vi "FileConfigDTOFromNative.vi"(8 "error in (no error)":errorcluster, 11 "FileConfig":T1={"rootFolder"=path "", "maxFileSize"=-1, "maxFileCount"=-1, "baseName"="", "extension"="", "delimiter"="", "calendarFolderTree"=FALSE}) -> (0 "error out":errorcluster, 3 "FileConfigDTO":T2={"rootFolder"="", "maxFileSize"=-1, "maxFileCount"=-1, "baseName"="", "extension"="", "delimiter"="", "calendarFolderTree"=FALSE})   [LabVIEW 2026, in "Lumberjack.lvlib"]
uses:
  Lumberjack.lvlib
  TypeDefs/ConfigDTO/FileConfigDTO.ctl
  TypeDefs/FileConfig.ctl
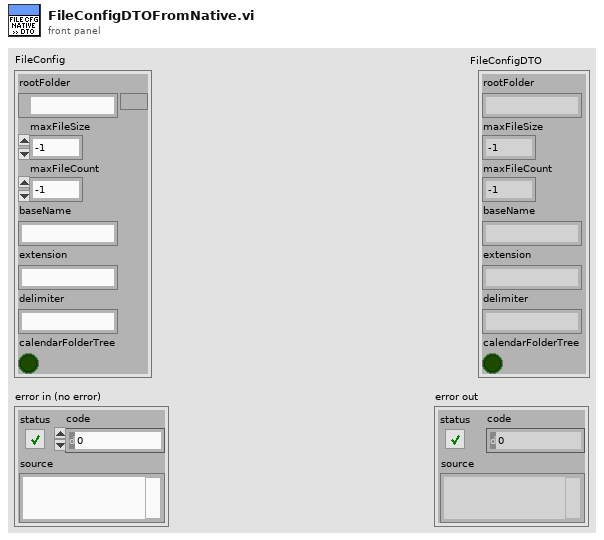
[diagram p1: front panel]
types:
  T1 = typedef "Lumberjack.lvlib/FileConfig.ctl" = cluster{"rootFolder":path, "maxFileSize":i64, "maxFileCount":i32, "baseName":string, "extension":string, "delimiter":string, "calendarFolderTree":bool}
  T2 = typedef "Lumberjack.lvlib/FileConfigDTO.ctl" = cluster{"rootFolder":string, "maxFileSize":i64, "maxFileCount":i32, "baseName":string, "extension":string, "delimiter":string, "calendarFolderTree":bool}
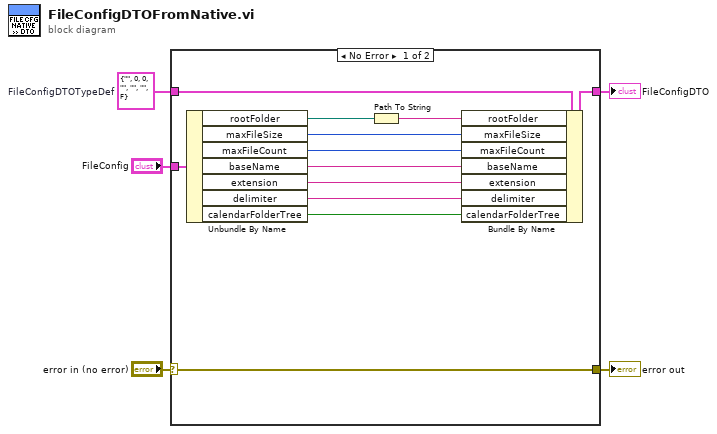
[diagram p0: block diagram]
diagram:
  w3 = T2 {"rootFolder"="", "maxFileSize"=0, "maxFileCount"=0, "baseName"="", "extension"="", "delimiter"="", "calendarFolderTree"=FALSE}  # FileConfigDTOTypeDef
  n1 = case shown="No Error" "error in (no error)" {
    selector: "error in (no error)" -> [w6 w19]
    tunnel: [w6 w19] -> w1
    tunnel: "FileConfig" -> [w16 _]
    tunnel: [w17 w18] -> w2
    tunnel: w3 -> [w15 w18]
    frame No Error {
      n2 = Unbundle By Name(w16) -> ("rootFolder"=w14:path, "maxFileSize"=w12:i64, "maxFileCount"=w11:i32, "baseName"=w10:string, "extension"=w9:string, "delimiter"=w8:string, "calendarFolderTree"=w7:bool)
      n3 = Path To String(path=w14) -> (string=w13:string)
      n4 = Bundle By Name(cluster=w15, "rootFolder"=w13, "maxFileSize"=w12, "maxFileCount"=w11, "baseName"=w10, "extension"=w9, "delimiter"=w8, "calendarFolderTree"=w7) -> (w17:T2)
    }
    frame Error {
    }
  }
  "error out" <- w1
  "FileConfigDTO" <- w2
